vi "Get_Initial_Displacements-2.vi"(3 "error IN":errorcluster, 4 "dR max":dbl, 5 "dR min":dbl, 6 "[IN] (X,Y)":dbl[][](array[numeric])) -> (0 "error OUT":errorcluster, 2 "[OUT] Raw Displacements":dbl[][](array[numeric]))   [LabVIEW 2013]
doc: "This subVI calculates raw frame-to-frame displacements (dX,dY)"
panel:
  out "# Displacements":i16
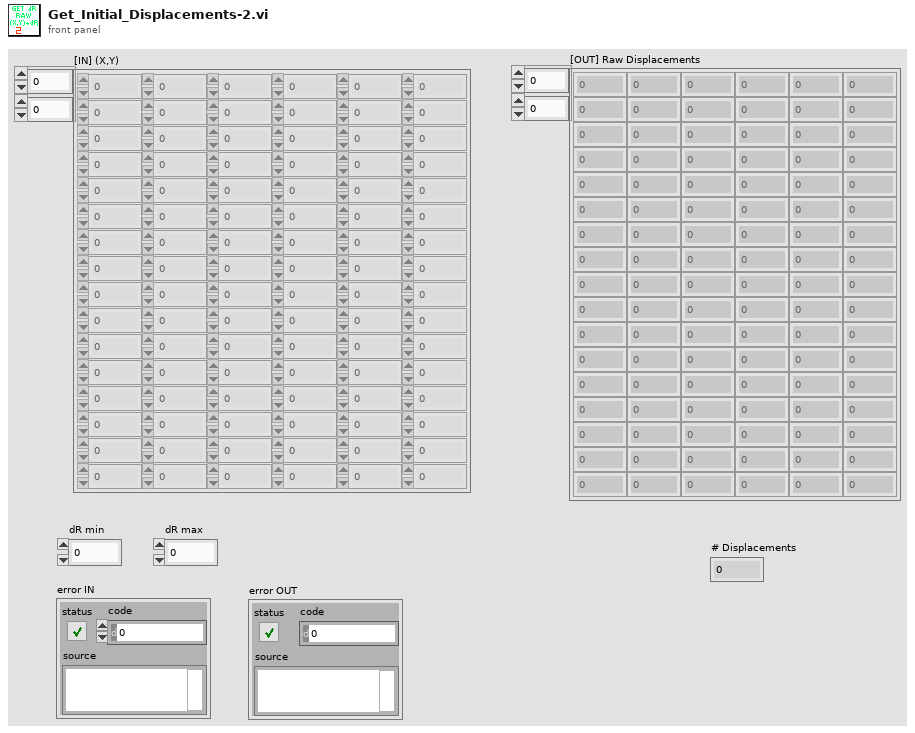
[diagram p1: front panel]
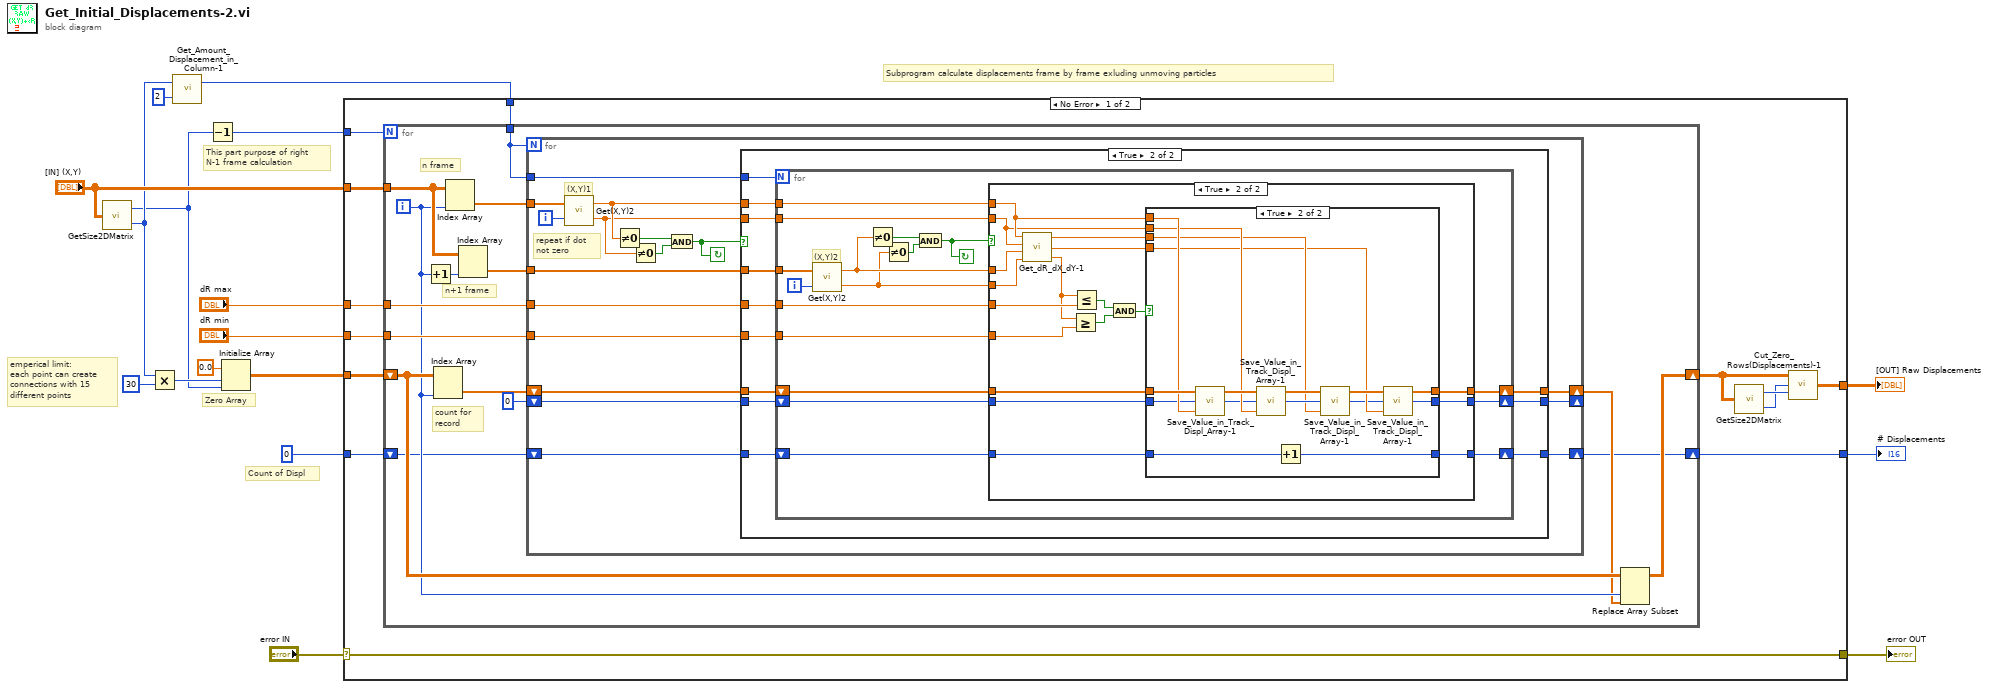
[diagram p0: block diagram]
diagram:
  # "emperical limit:\neach point can create \nconnections with 15 \ndifferent points"
  # "This part purpose of right\nN-1 frame calculation"
  # "Count of Displ"
  # "Subprogram calculate displacements frame by frame exluding unmoving particles"
  # "Zero Array"
  n1 = call "GetSize2DMatrix.vi"("Array IN (2D)"="[IN] (X,Y)") -> ("# Cols"=w5:i32, "# Rows"=w7:i32)
  n2 = Multiply(x=w7, y=30) -> (x*y=w15:i32)
  n3 = call "Get_Amount_Displacement_in_Column-1.vi"("multiplier"=2 ("y"), "# Rows"=w7) -> ("Displ amount"=w6:i32)  [unwired: 1 out]
  n4 = Decrement(x=w5) -> (x-1=w4:i32)
  n5 = Initialize Array(0.0 ("element"), w15, w5) -> (w13:dbl[][])
  n6 = case shown="No Error" "error IN" {
    selector: "error IN" -> [w18 w135]
    tunnel: "[IN] (X,Y)" -> [w30 _]
    tunnel: w13 -> [w29 w137]
    tunnel: "dR max" -> [w28 _]
    tunnel: "dR min" -> [w27 _]
    tunnel: [w23 w137] -> w10
    tunnel: i16 0 -> [w22 w136]
    tunnel: w6 -> [w21 _]
    tunnel: w4 -> [w20 _]
    tunnel: [w19 w136] -> w3
    tunnel: [w18 w135] -> w1
    frame No Error {
      n7 = for {
        N: w20 -> [_]
        tunnel: w30 -> [w45]
        shift-right: [w34] -> w24
        shift-left: w29 -> [w37]
        tunnel: w28 -> [w41]
        tunnel: w27 -> [w40]
        shift-right: [w32] -> w19
        shift-left: w22 -> [w33]
        tunnel: w21 -> [w31]
        i -> [w36]
        # "count for \nrecord"
        # "n+1 frame"
        # "n frame"
        n8 = Increment(x=w36) -> (x+1=w44:i32)
        n9 = Index Array(array=w37, index (col)=w36) -> (element=w39:dbl[])  [unwired: 1 in]
        n10 = Index Array(array=w45, index (col)=w36) -> (element=w43:dbl[])  [unwired: 1 in]
        n11 = Index Array(array=w45, index (col)=w44) -> (element=w42:dbl[])  [unwired: 1 in]
        n12 = for {
          N: w31 -> [_]
          tunnel: w43 -> [w52]
          tunnel: w31 -> [w62]
          tunnel: w42 -> [w61]
          tunnel: w41 -> [w60]
          tunnel: w40 -> [w59]
          shift-right: [w56] -> w35
          shift-left: w39 -> [w58]
          shift-right: [w55] -> _
          shift-left: 0 -> [w57]
          shift-right: [w53] -> w32
          shift-left: w33 -> [w54]
          i -> [w51]
          stop <- w46 continue-if-true
          # "repeat if dot \nnot zero"
          # "(X,Y)1"
          n13 = call "Get(X,Y)2.vi"("[IN] index of (X,Y)"=w51, "[IN] Array coordi\nnates (X,Y) in Frame"=w52) -> ("[OUT] Y"=w49:dbl, "[OUT] X"=w50:dbl)
          n14 = Not Equal To 0?(x=w50) -> (x != 0?=w48:bool)
          n15 = Not Equal To 0?(x=w49) -> (x != 0?=w47:bool)
          n16 = And(x=w48, y=w47) -> (x .and. y?=w46:bool)
          n17 = case shown="True" w46 {
            tunnel: w62 -> [_ w77]
            tunnel: w61 -> [_ w76]
            tunnel: w60 -> [_ w75]
            tunnel: w59 -> [_ w74]
            tunnel: w58 -> [w65 w73]
            tunnel: w57 -> [w64 w72]
            tunnel: [w65 w71] -> w56
            tunnel: [w64 w70] -> w55
            tunnel: w54 -> [w63 w69]
            tunnel: [w63 w68] -> w53
            tunnel: w50 -> [_ w67]
            tunnel: w49 -> [_ w66]
            frame False {
            }
            frame True {
              n18 = for {
                N: w77 -> [_]
                tunnel: w67 -> [w94]
                tunnel: w66 -> [w93]
                tunnel: w76 -> [w85]
                tunnel: w75 -> [w92]
                tunnel: w74 -> [w91]
                shift-right: [w88] -> w71
                shift-left: w73 -> [w90]
                shift-right: [w78] -> w70
                shift-left: w72 -> [w89]
                shift-right: [w86] -> w68
                shift-left: w69 -> [w87]
                i -> [w84]
                stop <- w79 continue-if-true
                # "(X,Y)2"
                n19 = call "Get(X,Y)2.vi"("[IN] index of (X,Y)"=w84, "[IN] Array coordi\nnates (X,Y) in Frame"=w85) -> ("[OUT] Y"=w80:dbl, "[OUT] X"=w81:dbl)
                n20 = Not Equal To 0?(x=w81) -> (x != 0?=w83:bool)
                n21 = Not Equal To 0?(x=w80) -> (x != 0?=w82:bool)
                n22 = And(x=w83, y=w82) -> (x .and. y?=w79:bool)
                n23 = case shown="True" w79 {
                  tunnel: w94 -> [_ w109]
                  tunnel: w93 -> [_ w108]
                  tunnel: w81 -> [_ w107]
                  tunnel: w80 -> [_ w106]
                  tunnel: w92 -> [_ w115]
                  tunnel: w91 -> [_ w113]
                  tunnel: w90 -> [w97 w105]
                  tunnel: w89 -> [w95 w104]
                  tunnel: [w97 w101] -> w88
                  tunnel: w87 -> [w96 w100]
                  tunnel: [w96 w99] -> w86
                  tunnel: [w95 w98] -> w78
                  frame False {
                  }
                  frame True {
                    n24 = call "Get_dR_dX_dY-1.vi"("Y2"=w106, "X2"=w107, "Y1"=w108, "X1"=w109) -> ("dR"=w114:dbl, "dY"=w102:dbl, "dX"=w103:dbl)
                    n25 = Greater Or Equal?(x=w114, y=w113) -> (x >= y?=w111:bool)
                    n26 = Less Or Equal?(x=w114, y=w115) -> (x <= y?=w112:bool)
                    n27 = And(x=w112, y=w111) -> (x .and. y?=w110:bool)
                    n28 = case shown="True" w110 {
                      tunnel: w109 -> [_ w131]
                      tunnel: w108 -> [_ w128]
                      tunnel: w105 -> [w118 w132]
                      tunnel: w104 -> [w116 w130]
                      tunnel: w103 -> [_ w124]
                      tunnel: w102 -> [_ w122]
                      tunnel: [w118 w120] -> w101
                      tunnel: w100 -> [w117 w134]
                      tunnel: [w117 w133] -> w99
                      tunnel: [w116 w119] -> w98
                      frame False {
                      }
                      frame True {
                        n29 = call "Save_Value_in_Track_Displ_Array-1.vi"("[IN] Value"=w131, "[IN] Index"=w130, "[IN] Empty tracks\nfor points saving"=w132) -> ("[OUT] Index ++"=w127:i32, "[OUT Track with saved value"=w129:dbl[])  [unwired: 1 in]
                        n30 = call "Save_Value_in_Track_Displ_Array-1.vi"("[IN] Value"=w128, "[IN] Index"=w127, "[IN] Empty tracks\nfor points saving"=w129) -> ("[OUT] Index ++"=w125:i32, "[OUT Track with saved value"=w126:dbl[])  [unwired: 1 in]
                        n31 = Increment(x=w134) -> (x+1=w133:i16)
                        n32 = call "Save_Value_in_Track_Displ_Array-1.vi"("[IN] Value"=w124, "[IN] Index"=w125, "[IN] Empty tracks\nfor points saving"=w126) -> ("[OUT] Index ++"=w121:i32, "[OUT Track with saved value"=w123:dbl[])  [unwired: 1 in]
                        n33 = call "Save_Value_in_Track_Displ_Array-1.vi"("[IN] Value"=w122, "[IN] Index"=w121, "[IN] Empty tracks\nfor points saving"=w123) -> ("[OUT] Index ++"=w119:i32, "[OUT Track with saved value"=w120:dbl[])  [unwired: 1 in]
                      }
                    }
                  }
                }
              }
            }
          }
        }
        n34 = Replace Array Subset(array=w37, new element=w35, index (col)=w36) -> (w34:dbl[][])  [unwired: 1 in]
      }
      n35 = call "GetSize2DMatrix.vi"("Array IN (2D)"=w24) -> ("# Cols"=w26:i32, "# Rows"=w25:i32)
      n36 = call "Cut_Zero_Rows(Displacements)-1.vi"("# Cols"=w26, "# Rows"=w25, "Array IN"=w24) -> ("Array OUT"=w23:dbl[][])
    }
    frame Error {
    }
  }
  "error OUT" <- w1
  "[OUT] Raw Displacements" <- w10
  "# Displacements" <- w3
